vi "get file properties.vi"(6 "File Property Indeces":i32[](array[numeric]), 8 "error in":errorcluster, 10 "dictionary":T1, 11 "data table in":T2) -> (0 "error out":errorcluster, 1 "File Property Values":string[](array[string]), 2 "File Property Names":string[](array[string]), 3 "Data table out":T2)   [LabVIEW 2015, in "TDMS datalogger runtime.lvclass"]
uses:
  TDMS datalogger runtime.lvclass
  <vilib>/NI/Tag Bus/table/data table.ctl
  <vilib>/NI/Tag Bus/dictionary/full data dictionary.ctl
  <vilib>/NI/Tag Bus/table/data polymorphs/read one/read String.vi
  <vilib>/NI/Tag Bus/table/data table.lvlib
  <vilib>/NI/Tag Bus/dictionary/data dictionary.lvclass
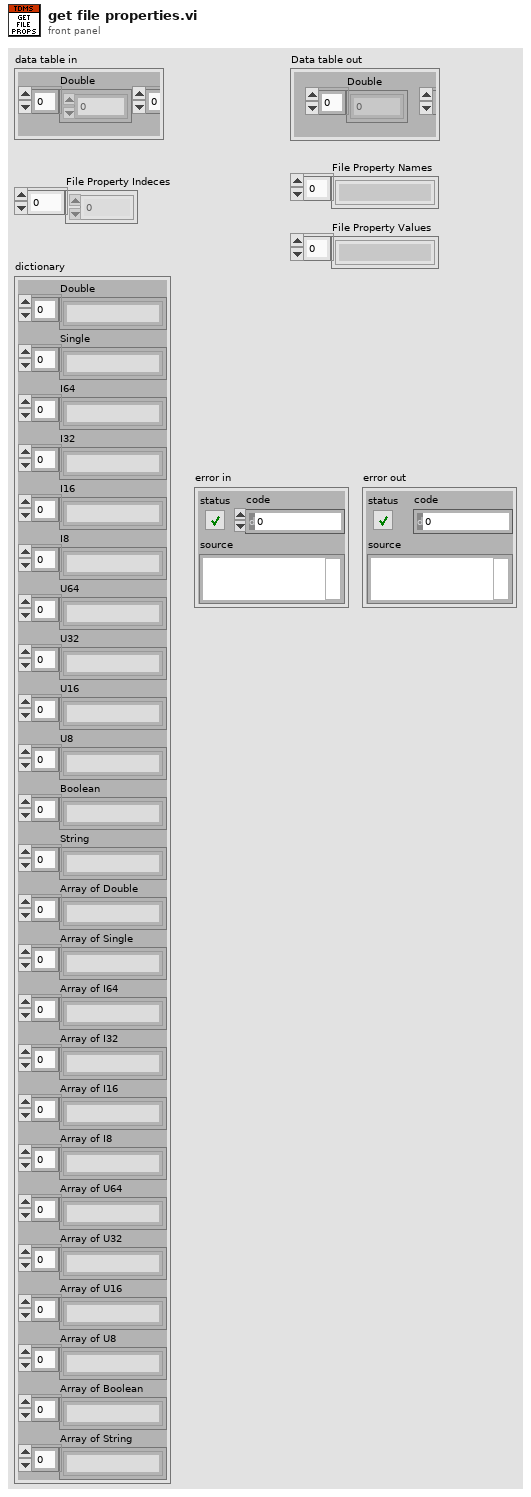
[diagram p1: front panel]
types:
  T1 = typedef "tag bus.lvlib/data dictionary.lvclass/full data dictionary.ctl" = cluster{"Double":string[], "Single":string[], "I64":string[], "I32":string[], "I16":string[], "I8":string[], "U64":string[], "U32":string[], "U16":string[], "U8":string[], "Boolean":string[], "String":string[], "Array of Double":string[], "Array of Single":string[], "Array of I64":string[], "Array of I32":string[], "Array of I16":string[], "Array of I8":string[], "Array of U64":string[], "Array of U32":string[], "Array of U16":string[], "Array of U8":string[], "Array of Boolean":string[], "Array of String":string[]}
  T2 = typedef "tag bus.lvlib/data table.lvlib/data table.ctl" = cluster{"Double":dbl[], "Single":sgl[], "I64":i64[], "I32":i32[], "I16":i16[], "I8":i8[], "U64":u64[], "U32":u32[], "U16":u16[], "U8":u8[], "Boolean":bool[], "String":string[], "Array of Double":cluster{"DBL Array":dbl[]}[], "Array of Single":cluster{"SGL Array":sgl[]}[], "Array of I64":cluster{"I64 Array":i64[]}[], "Array of I32":cluster{"I32 Array":i32[]}[], "Array of I16":cluster{"I16 Array":i16[]}[], "Array of I8":cluster{"I8 Array":i8[]}[], "Array of U64":cluster{"U64 Array":u64[]}[], "Array of U32":cluster{"U32 Array":u32[]}[], "Array of U16":cluster{"U16 Array":u16[]}[], "Array of U8":cluster{"U8 Array":u8[]}[], "Array of Boolean":cluster{"Boolean Array":bool[]}[], "Array of String":cluster{"String Array":string[]}[]}
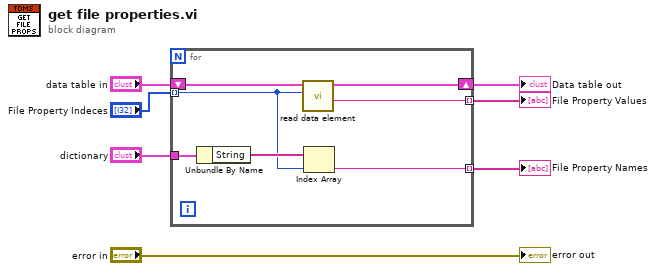
[diagram p0: block diagram]
diagram:
  n1 = for {
    tunnel: "File Property Indeces" -> [w9] mode=indexing
    shift-right: [w13] -> w5
    shift-left: "data table in" -> [w14]
    tunnel: [w12] -> w4 mode=indexing
    tunnel: "dictionary" -> [w11]
    tunnel: [w8] -> w2 mode=indexing
    n2 = Unbundle By Name(w11) -> ("String"=w10:string[])
    n3 = call-poly <vilib>:"read data element.vi"("index"=w9, "data table in"=w14) -> ("value"=w12:string, "data table out"=w13:T2)  [unwired: 8 in]
    n4 = Index Array(array=w10, index=w9) -> (element=w8:string)
  }
  "Data table out" <- w5
  "File Property Values" <- w4
  "File Property Names" <- w2
  "error out" <- "error in"
